vi "Read value elevator location.vi"(8 "error in (no error)":errorcluster, 11 "Sim Display Console Actor in":refnum<class "Sim Display Console Actor.lvclass">) -> (0 "error out":errorcluster, 3 "Sim Display Console Actor out":refnum<class "Sim Display Console Actor.lvclass">)   [LabVIEW 2019, in "Simulated Display Console Actor.lvlib" / "Sim Display Console Actor.lvclass"]
uses:
  Sim Display Console Actor.lvclass
  Elevator Controller/Elevator Controller Actor Messages/Wait for First Request Msg/Wait for First Request Msg.lvclass
  <vilib>/ActorFramework/Actor/Actor.lvclass
  Elevator Controller/Elevator Controller Actor Messages/Match Elevator Position and Location Msg/Match Elevator Position and Location Msg.lvclass
  C:/Workspace/CLA/Elevator AF 2nd/Dsiplay Console Actor/Dsiplay Console Actor/Dsiplay Console Actor.lvclass
  C:/Program Files (x86)/National Instruments/LabVIEW 2019/vi.lib/ActorFramework/Actor/Actor.lvclass
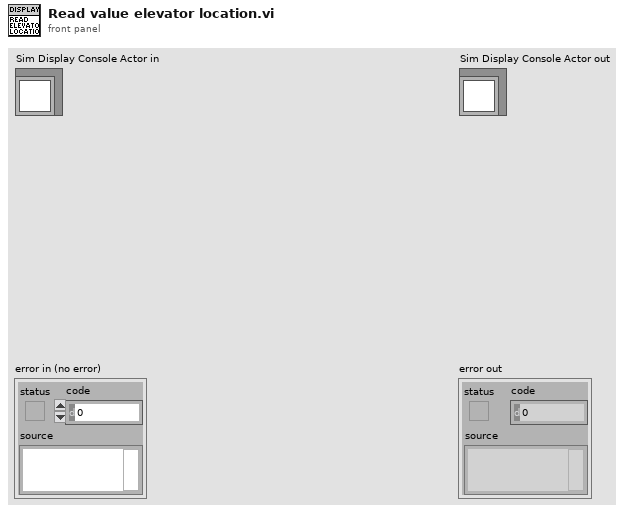
[diagram p1: front panel]
types:
  T1 = typedef "Simulated Display Console Actor.lvlib/Sim Display Console Actor.lvclass/Floor -Enum.ctl" = enum16{"First Floor", "Send Floor", "Third Floor", "Fourth Floor"}
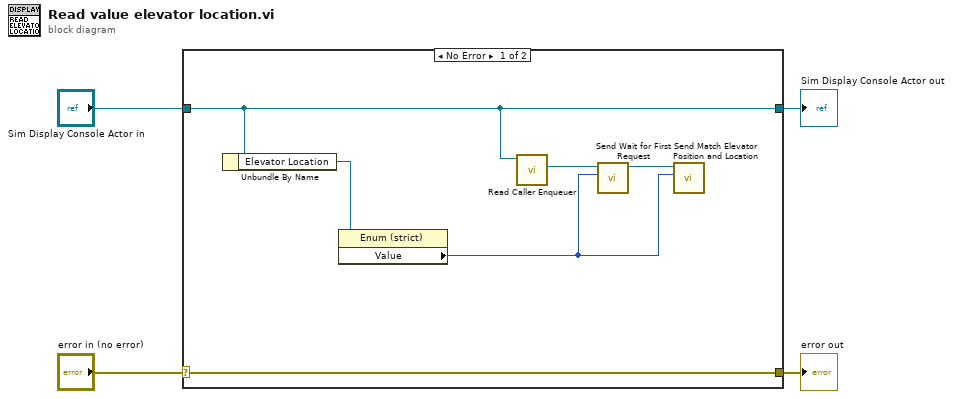
[diagram p0: block diagram]
diagram:
  n1 = case shown="No Error" "error in (no error)" {
    selector: "error in (no error)" -> [w10 w12]
    tunnel: [w10 w12] -> w3
    tunnel: [w8 w11] -> w1
    tunnel: "Sim Display Console Actor in" -> [w8 w11]
    frame No Error {
      n2 = Unbundle By Name(w8) -> ("Elevator Location"=w9:refnum<vi>)
      n3 = property class="Enum (strict)"(reference=w9) -> ("Value"=w5:T1)  [unwired: 1 in, 2 out]
      n4 = call <vilib>:"Read Caller Enqueuer.vi"("Actor"=w8) -> ("Caller Enqueuer"=w7:refnum<class "Message Enqueuer.lvclass">)  [unwired: 10 in]
      n5 = call "Send Wait for First Request.vi"("Elevator Location"=w5, "Message Enqueuer"=w7) -> ("Message Enqueuer out"=w6:refnum<class "Message Enqueuer.lvclass">)  [unwired: 8 in, 1 out]
      n6 = call "Send Match Elevator Position and Location.vi"("Elevator Position"=w5, "Message Enqueuer"=w6) -> ()  [unwired: 8 in, 2 out]
    }
    frame Error {
    }
  }
  "error out" <- w3
  "Sim Display Console Actor out" <- w1
